vi "Do.vi"(8 "error in (no error)":errorcluster, 10 "Actor in":refnum<class "Actor.lvclass">, 11 "Update PV":refnum<class "Update PV.lvclass">) -> (0 "error out":errorcluster, 2 "Actor out":refnum<class "Actor.lvclass">)   [LabVIEW 2014, in "CS++DeviceGUIActor.lvlib" / "Update PV.lvclass"]
doc: "(<B>Filename</B>: Actor Framework.lvlib:Message.lvclass:Do.vi)\n\nDefines what a message does when it is received by an actor. Generally, a message instructs an actor to invoke one of its methods.\n\nBy default, this method does nothing. A child class must override it to define behavior. Create a child class by using the Actor Framework Message Maker dialog box."
uses:
  Update PV.lvclass
  <vilib>/ActorFramework/Actor/Actor.lvclass
  CS++DeviceGUIActor/CS++DeviceGUIActor.lvclass
  CS++PVMonitor Messages/CS++PVUpdate Msg/CS++PVUpdate Msg.lvclass/CS++PVUpdate Msg.ctl
  Classes/CS++ProcessVariables/ProcessVariable/PV.lvclass
  CS++PVMonitor Messages/CS++PVUpdate Msg/CS++PVUpdate Msg.lvclass
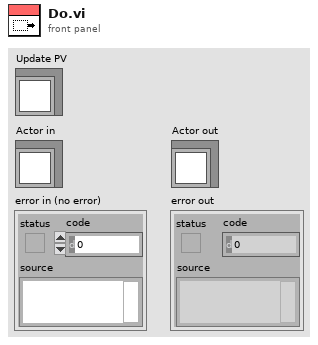
[diagram p1: front panel]
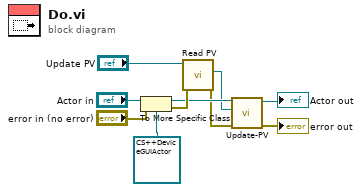
[diagram p0: block diagram]
diagram:
  n1 = To More Specific Class(target class=refnum<class "CS++DeviceGUIActor.lvclass"> refnum ("CS++DeviceGUIActor.lvlib:CS++DeviceGUIActor.lvclass"), reference="Actor in", error in="error in (no error)") -> (specific class reference=w5:refnum<class "CS++DeviceGUIActor.lvclass">, error out=w7:errorcluster)
  n2 = call "Read PV.vi"("error in (no error)"=w7, "CS++PVUpdate Msg in"="Update PV") -> ("error out"=w3:errorcluster, "PV"=w4:refnum<class "PV.lvclass">)  [unwired: 7 in, 1 out]
  n3 = call "Update-PV.vi"("Error In"=w3, "PV"=w4, "CS++DeviceGUIActor in"=w5) -> ("Error Out"=→"error out":errorcluster, "CS++DeviceGUIActor out"=→"Actor out":refnum<class "CS++DeviceGUIActor.lvclass">)  [unwired: 7 in]
